vi "Get Recipe Status.vi"(8 "error in (no error)":errorcluster, 11 "Recipe Status in":refnum<class "Recipe Status.lvclass">) -> (0 "error out":errorcluster, 2 "Recipe State Data":refnum<data-value>, 3 "Recipe Status out":refnum<class "Recipe Status.lvclass">)   [LabVIEW 2022 SP3, in "Recipe Status.lvclass"]
uses:
  Recipe Status.lvclass
  Recipe State Data/Recipe State Data.lvclass
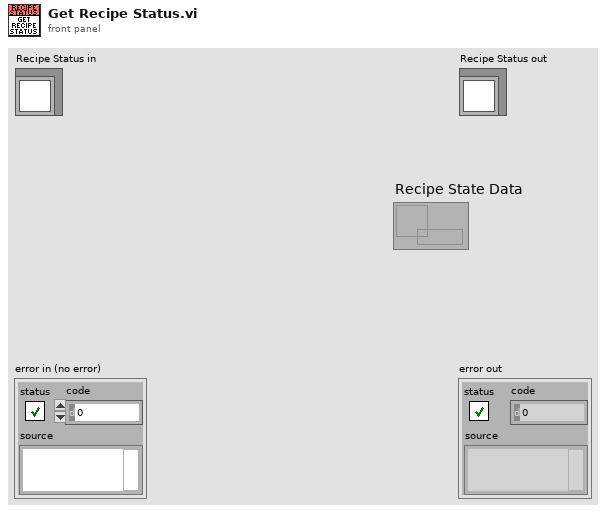
[diagram p1: front panel]
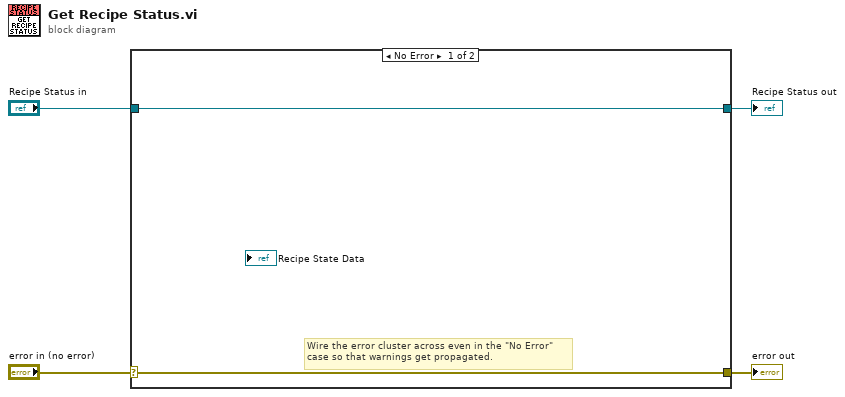
[diagram p0: block diagram]
diagram:
  n1 = case shown="No Error" "error in (no error)" {
    selector: "error in (no error)" -> [w5 w8]
    tunnel: [w5 w8] -> w3
    tunnel: [w6 w7] -> w1
    tunnel: "Recipe Status in" -> [w6 w7]
    frame No Error {
      # "Wire the error cluster across even in the \"No Error\"\ncase so that warnings get propagated."
    }
    frame Error {
    }
  }
  "error out" <- w3
  "Recipe Status out" <- w1
